vi "CRYUpdate Unicode Tree Headers.vi"(6 "Caption":string, 7 "Interpret as Unicode (T)":bool=TRUE, 8 "error in (no error)":errorcluster, 9 "Row Headers[]":string[](array[string]), 10 "Column Headers[]":string[](array[string]), 11 "Tree Ref":refnum<vi>) -> (0 "error out":errorcluster, 3 "Tree Ref":refnum<vi>)   [LabVIEW 2013]
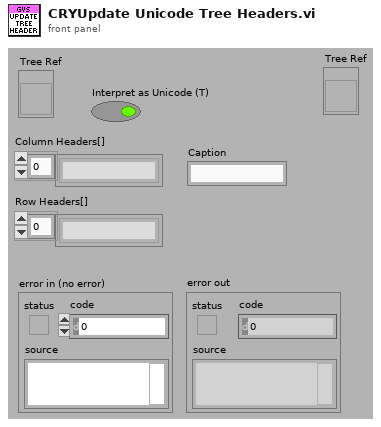
[diagram p1: front panel]
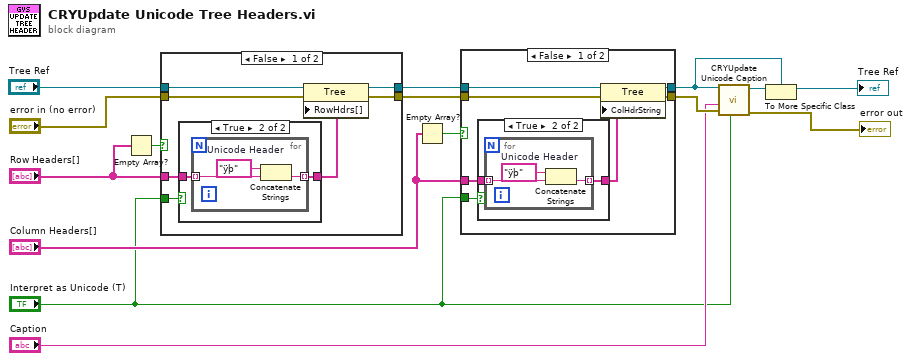
[diagram p0: block diagram]
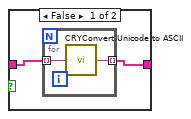
[diagram p2: hidden frame]
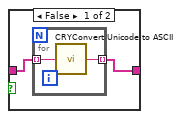
[diagram p4: hidden frame]
diagram:
  n1 = Empty Array?(array="Row Headers[]") -> (empty?=w13:bool)
  n2 = case shown="False" w13 {
    tunnel: "Row Headers[]" -> [w22 _]
    tunnel: "Tree Ref" -> [w20 w33]
    tunnel: "error in (no error)" -> [w19 w32]
    tunnel: [w18 w33] -> w14
    tunnel: "Interpret as Unicode (T)" -> [w17 _]
    tunnel: [w16 w32] -> w9
    frame False {
      n3 = case shown="True" w17 {
        tunnel: w22 -> [w24 w28]
        tunnel: [w23 w27] -> w21
        frame False {
          n4 = for {
            tunnel: w24 -> [w26] mode=indexing
            tunnel: [w25] -> w23 mode=indexing
            n5 = call "CRYConvert Unicode to ASCII.vi"("Unicode"=w26) -> ("ASCII"=w25:string)  [unwired: 4 in]
          }
        }
        frame True {
          n6 = for {
            tunnel: w28 -> [w31] mode=indexing
            tunnel: [w30] -> w27 mode=indexing
            w29 = "ÿþ"  # Unicode Header
            n7 = Concatenate Strings(w29, w31) -> (w30:string)
          }
        }
      }
      n8 = property class="Tree"(reference=w20, error in=w19, "RowHdrs[]"=w21) -> (reference out=w18:refnum<vi>, error out=w16:errorcluster)
    }
    frame True {
    }
  }
  n9 = Empty Array?(array="Column Headers[]") -> (empty?=w10:bool)
  n10 = case shown="False" w10 {
    tunnel: "Column Headers[]" -> [w40 _]
    tunnel: [w39 w51] -> w8
    tunnel: w9 -> [w37 w51]
    tunnel: w14 -> [w36 w50]
    tunnel: "Interpret as Unicode (T)" -> [w35 _]
    tunnel: [w34 w50] -> w5
    frame False {
      n11 = case shown="True" w35 {
        tunnel: w40 -> [w42 w46]
        tunnel: [w41 w45] -> w38
        frame False {
          n12 = for {
            tunnel: w42 -> [w44] mode=indexing
            tunnel: [w43] -> w41 mode=indexing
            n13 = call "CRYConvert Unicode to ASCII.vi"("Unicode"=w44) -> ("ASCII"=w43:string)  [unwired: 4 in]
          }
        }
        frame True {
          n14 = for {
            tunnel: w46 -> [w49] mode=indexing
            tunnel: [w48] -> w45 mode=indexing
            w47 = "ÿþ"  # Unicode Header
            n15 = Concatenate Strings(w47, w49) -> (w48:string)
          }
        }
      }
      n16 = property class="Tree"(reference=w36, error in=w37, "ColHdrString"=w38) -> (reference out=w34:refnum<vi>, error out=w39:errorcluster)
    }
    frame True {
    }
  }
  n17 = call "CRYUpdate Unicode Caption.vi"("Interpret as Unicode (T)"="Interpret as Unicode (T)", "error in (no error)"=w8, "Caption"="Caption", "Control Reference"=w5) -> ("error out"=→"error out":errorcluster, "Control Reference"=w6:refnum<vi>)  [unwired: 4 in]
  n18 = To More Specific Class(target class=w5, reference=w6) -> (specific class reference=→"Tree Ref":refnum<vi>)  [unwired: 1 in, 1 out]
